vi "Configure VIP Publish.vi"(8 "error in (no error)":errorcluster, 10 "JSON string":string) -> (0 "error out":errorcluster, 3 "VIP Publish out":refnum<class "VIP Publish.lvclass">)   [LabVIEW 2014, in "VIP Publish.lvclass"]
uses:
  VIP Publish.lvclass
  Shared/Controls/VIP Publish - STYP.ctl
  VIP Publish.lvclass/VIP Publish.ctl
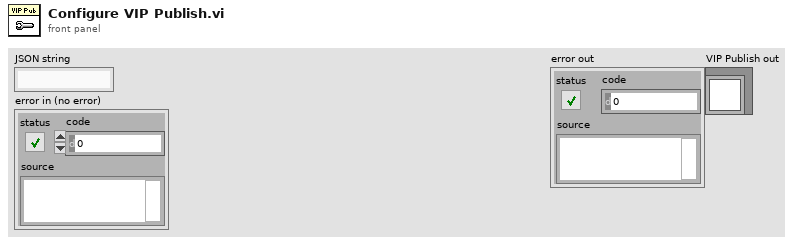
[diagram p1: front panel]
types:
  T1 = typedef "VIP Publish - STYP.ctl" = cluster{"VIP Path":string, "Repo Name":string}
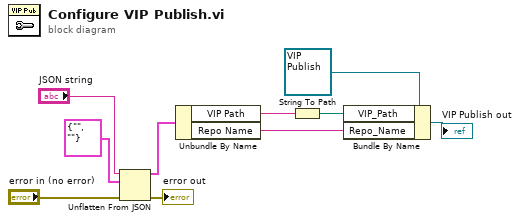
[diagram p0: block diagram]
diagram:
  n1 = Unflatten From JSON(JSON string="JSON string", type and defaults=T1 {"VIP Path"="", "Repo Name"=""} ("VIP Publish"), error in (no error)="error in (no error)") -> (value=w6:T1, error out=→"error out":errorcluster)  [unwired: 4 in]
  n2 = Unbundle By Name(w6) -> ("VIP Path"=w4:string, "Repo Name"=w1:string)
  n3 = String To Path(string=w4) -> (path=w3:path)
  n4 = Bundle By Name(cluster=refnum<class "VIP Publish.lvclass"> refnum ("VIPB Build out"), "VIP_Path"=w3, "Repo_Name"=w1) -> (→"VIP Publish out":refnum<class "VIP Publish.lvclass">)
